vi "Configure Surge-Drop Continuous Mode.vi"(0 "VISA resource name":refnum<visa-resource-name>, 5 "Enable  Continuous Surge Drop (F:Disable)":bool, 11 "error in (no error)":errorcluster) -> (4 "VISA resource name out":refnum<visa-resource-name>, 15 "error out":errorcluster)   [LabVIEW 2020, in "eec 6700.lvlib"]
doc: "Enables or Disables the <B>Continuous Surge Drop</B> in the power source instrument.\n\n<B>Range</B> : [Disable, Enable]\n\nThe Surge Drop-Continuous parameter setting configures whether the surge or drop voltage will occur continuously for each size wave of the test routine. The operator has the choice of selecting Enable or Disable. If the Surge Drop-Continuous parameter is selected Disable the surge or drop voltage will occur only on the first sine wave and will not repeat on any other sine waves unless the trigger soft key is pressed."
uses:
  <instrlib>/EEC6700LV-driver/eec 6700.lvlib
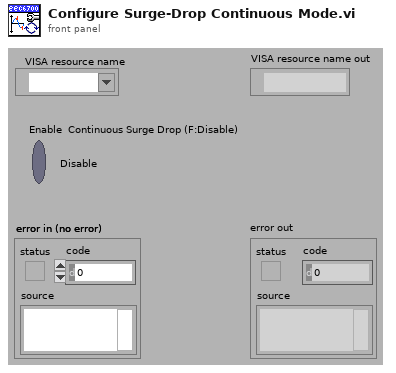
[diagram p1: front panel]
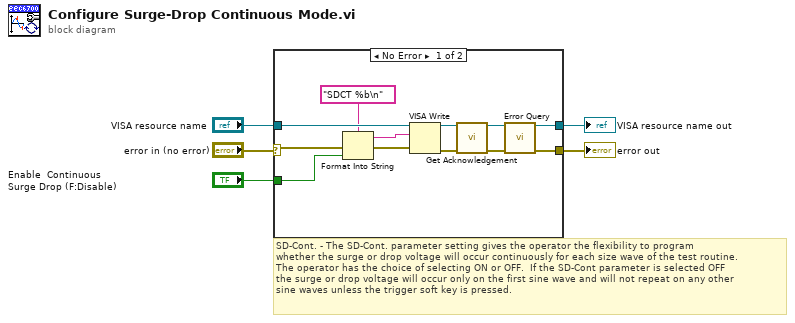
[diagram p0: block diagram]
diagram:
  # "SD-Cont. - The SD-Cont. parameter setting gives the operator the flexibility to program \nwhether the surge or drop voltage will occur continuously for each size wave of the test routine.  \nThe operator has the choice of selecting ON or OFF.  If the SD-Cont parameter is selected OFF \nthe surge or drop voltage will occur only on the first sine wave and will not repeat on any other \nsine waves unless the trigger soft key is pressed."
  n1 = case shown="No Error" "error in (no error)" {
    selector: "error in (no error)" -> [w12 w19]
    tunnel: "VISA resource name" -> [w17 w18]
    tunnel: [w14 w18] -> w4
    tunnel: [w13 w19] -> w3
    tunnel: "Enable  Continuous Surge Drop (F:Disable)" -> [w10 _]
    frame No Error {
      n2 = Format Into String(format string="SDCT %b\n" ("Command"), error in=w12, w10) -> (resulting string=w16:string, error out=w11:errorcluster)  [unwired: 1 in]
      n3 = VISA Write(VISA resource name=w17, write buffer=w16, error in (no error)=w11) -> (VISA resource name out=w6:refnum<visa-resource-name>, error out=w9:errorcluster)  [unwired: 1 out]
      n4 = call <instrlib>:"Get Acknowledgement.vi"("VISA resource name"=w6, "error in (no error)"=w9) -> ("VISA resource name out"=w7:refnum<visa-resource-name>, "error out"=w8:errorcluster)  [unwired: 12 in]
      n5 = call <instrlib>:"Error Query.vi"("VISA resource name"=w7, "error in (no error)"=w8) -> ("VISA resource name out"=w14:refnum<visa-resource-name>, "error out"=w13:errorcluster)  [unwired: 10 in, 2 out]
    }
    frame Error {
    }
  }
  "error out" <- w3
  "VISA resource name out" <- w4
